vi "camera test.vi"() -> ()   [LabVIEW 2019]
uses:
  <vilib>/userDefined/High Color/IMAQdx.ctl
  <vilib>/vision/NI_Vision_Development_Module.lvlib
  defectsWrapper/defectsWrapper.lvlib
  <vilib>/vision/driver/NI_Vision_Acquisition_Software.lvlib
panel:
  out "Pallet Defects View":T1(plugin-control)
  out "size":dbl=5.0
  in  "threshoulds":dbl[](array[numeric])=[900.0, 1000.0, 1600.0, 2400.0, 3000.0, 3000.0]
  in  "Boolean":bool
  in  "stop ok":bool
  out "stop live view":bool
  out "error out 6":errorcluster
  out "LIVE VIEW":T1(plugin-control)
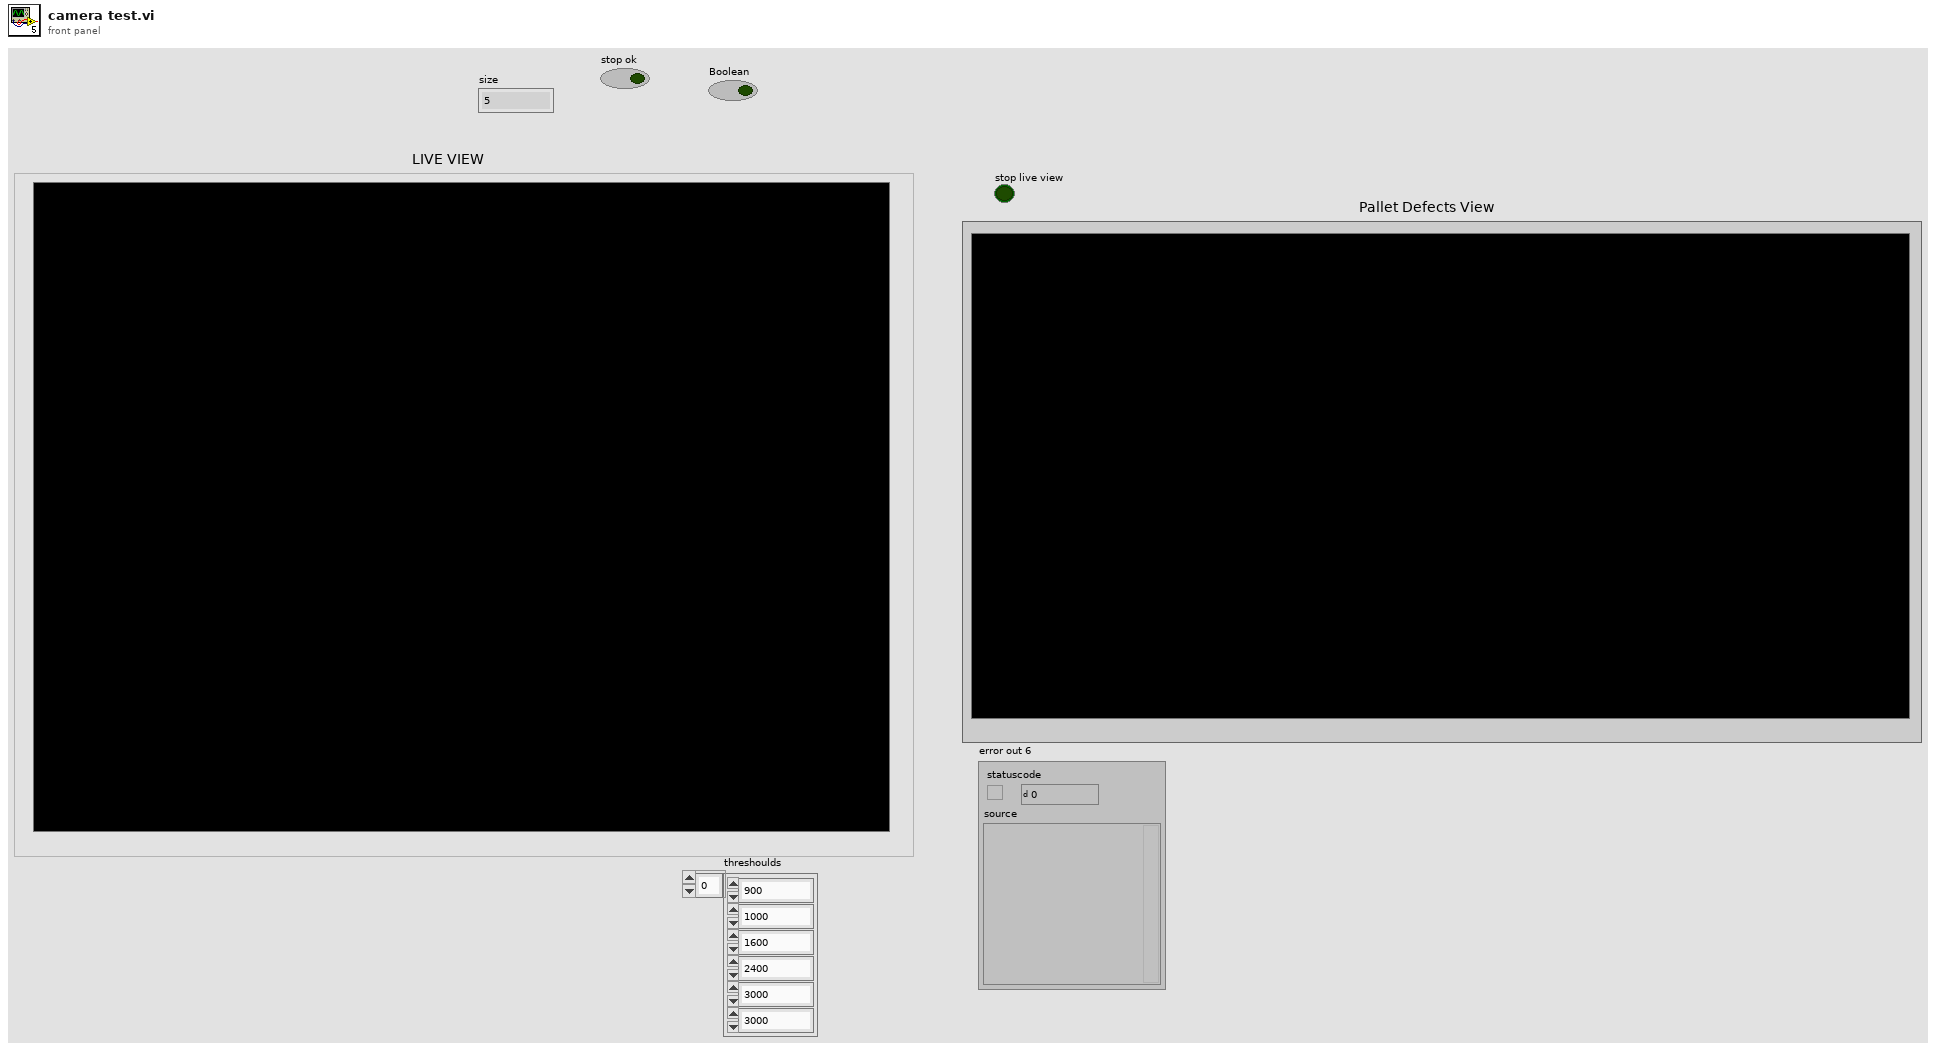
[diagram p1: front panel]
types:
  T1 = typedef "IMAQ Image.ctl" = refnum<image>
  T2 = typedef "IMAQdx.ctl" = refnum<k21>
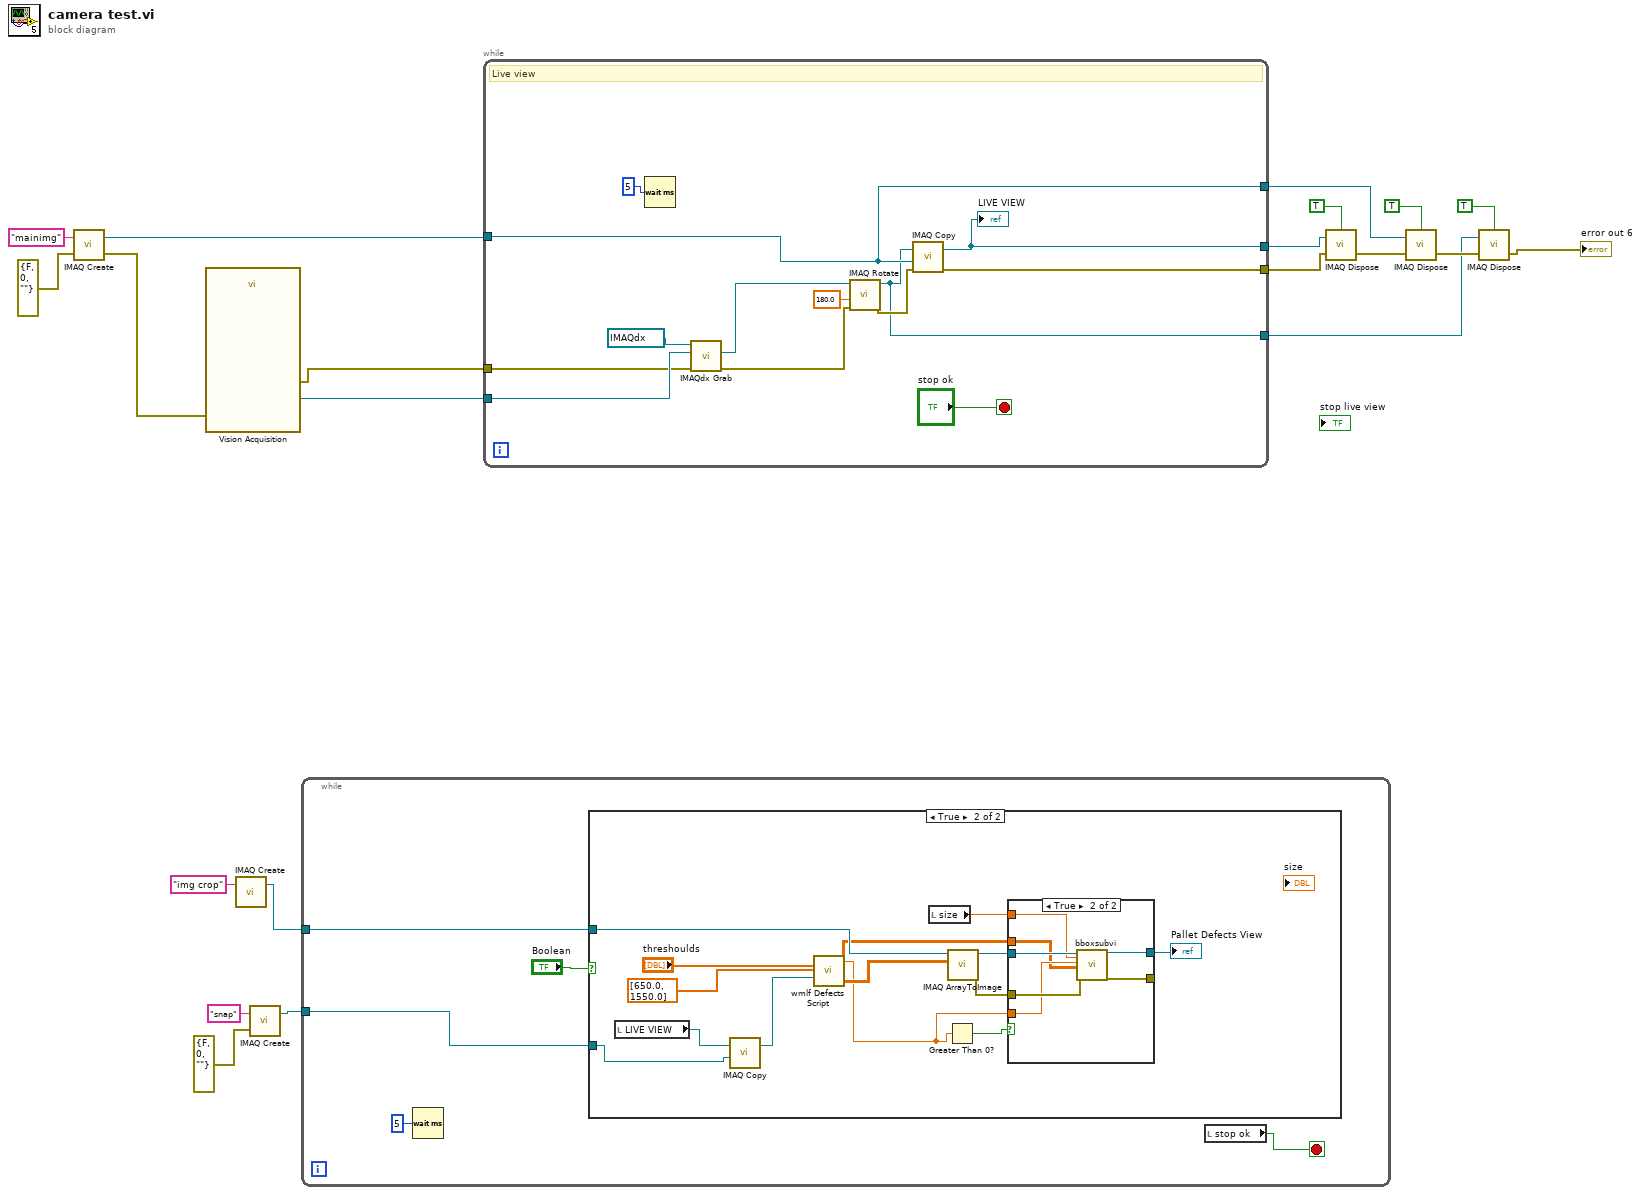
[diagram p0: block diagram]
diagram:
  n1 = call "IMAQ Create"("Image Name"="mainimg", "error in (no error)"=errorcluster {"status"=FALSE, "code"=0, "source"=""}) -> ("New Image"=w20:T1, "error out"=w2:errorcluster)  [unwired: 3 in]
  n2 = call "Vision Acquisition"("error in"=w2) -> ("Image Out"=w3:T1, "error out"=w1:errorcluster)  [unwired: 24 in, 1 out]
  n3 = call "IMAQ Create"("Image Name"="img crop") -> ("New Image"=w4:T1)  [unwired: 4 in, 1 out]
  n4 = call "IMAQ Create"("Image Name"="snap", "error in (no error)"=errorcluster {"status"=FALSE, "code"=0, "source"=""}) -> ("New Image"=w6:T1)  [unwired: 3 in, 1 out]
  n5 = while {
    tunnel: w6 -> [w25]
    tunnel: w4 -> [w24]
    stop <- w23 stop-if-true
    n6 = Wait (ms)(milliseconds to wait=u32 5) -> ()  [unwired: 1 out]
    n7 = case shown="True" "Boolean" {
      tunnel: w25 -> [_ w38]
      tunnel: w24 -> [_ w29]
      frame False {
      }
      frame True {
        n8 = local read "LIVE VIEW"() -> (w37:T1)
        n9 = call "IMAQ Copy"("Image Dst"=w38, "Image Src"=w37) -> ("Image Dst Out"=w36:T1)  [unwired: 4 in, 1 out]
        n10 = call "wmlf Defects Script.vi"("threshoulds"="threshoulds", "margin"=dbl[] [650.0, 1550.0], "Image 3"=w36) -> ("x-y defects locs"=w27:dbl[][], "defnum"=w28:dbl, "crop array"=w30:dbl[][])  [unwired: 16 in, 6 out]
        n11 = local read "size"() -> (w34:dbl)
        n12 = Greater Than 0?(x=w28) -> (x > 0?=w33:bool)
        n13 = call "IMAQ ArrayToImage"("Image Pixels (U8)"=w30, "Image"=w29) -> ("error out"=w32:errorcluster, "Image Out"=w31:T1)  [unwired: 8 in]
        n14 = case shown="True" w33 {
          tunnel: w31 -> [w41 w49]
          tunnel: w32 -> [w42 w48]
          tunnel: [w42 w47] -> _
          tunnel: [w41 w46] -> w35
          tunnel: w34 -> [_ w45]
          tunnel: w28 -> [_ w44]
          tunnel: w27 -> [_ w43]
          frame False {
          }
          frame True {
            n15 = call "bboxsubvi.vi"("Image"=w49, "size"=w45, "def num"=w44, "array"=w43, "error in"=w48) -> ("Image Out"=w46:T1, "error out"=w47:errorcluster)  [unwired: 13 in]
          }
        }
        "Pallet Defects View" <- w35
      }
    }
    n16 = local read "stop ok"() -> (w23:bool)
  }
  n17 = while {
    tunnel: w20 -> [w57]
    tunnel: [w59] -> w17
    tunnel: [w58] -> w16
    tunnel: [w57] -> w14
    tunnel: [w56] -> w11
    tunnel: w3 -> [w54]
    tunnel: w1 -> [w53]
    stop <- "stop ok" stop-if-true
    # "Live view"
    n18 = Wait (ms)(milliseconds to wait=u32 5) -> ()  [unwired: 1 out]
    n19 = call <vilib>:"IMAQdx Grab.vi"("error in"=w53, "Image In"=w54, "Session In"=T2 "cam0") -> ("error out"=w52:errorcluster, "Image Out"=w51:T1)  [unwired: 1 in, 6 out]
    n20 = call "IMAQ Rotate"("error in (no error)"=w52, "Angle (degrees)"=sgl 180.0, "Image Src"=w51) -> ("error out"=w61:errorcluster, "Image Dst Out"=w56:T1)  [unwired: 7 in]
    n21 = call "IMAQ Copy"("error in (no error)"=w61, "Image Dst"=w57, "Image Src"=w56) -> ("error out"=w58:errorcluster, "Image Dst Out"=w59:T1)  [unwired: 3 in]
    "LIVE VIEW" <- w59
  }
  n22 = call "IMAQ Dispose"("All Images? (No)"=TRUE, "Image"=w17, "error in (no error)"=w16) -> ("error out"=w15:errorcluster)  [unwired: 3 in]
  n23 = call "IMAQ Dispose"("All Images? (No)"=TRUE, "Image"=w14, "error in (no error)"=w15) -> ("error out"=w12:errorcluster)  [unwired: 3 in]
  n24 = call "IMAQ Dispose"("All Images? (No)"=TRUE, "Image"=w11, "error in (no error)"=w12) -> ("error out"=→"error out 6":errorcluster)  [unwired: 3 in]
